vi "sine_wave_generator.vi"(7 "Source":T1={"Source"=TRUE, "Source type"=FALSE, "Amplitude"=1.0, "Period"=100.0} {"Amplitude" scale=0.0..1.0; "Period" scale=1.0..1000.0}) -> (8 "Output":dbl)   [LabVIEW 2016]
doc: "Use this VI to generate sine wave.\n\nInputs:\nSource (typedef).\nOutputs:\nOutput.\n\nMuhannad Alghamdi\nCSUSB Physics 350"
uses:
  typedefs/periodic_signal_control.ctl
panel:
  out "Call counter":dbl
  # "Sine Wave Generator"
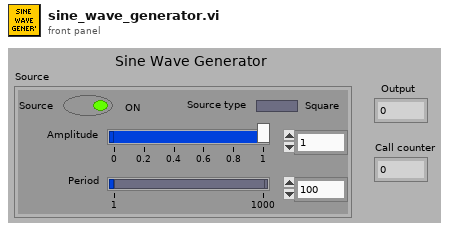
[diagram p1: front panel]
types:
  T1 = typedef "periodic_signal_control.ctl" = cluster{"Source":bool, "Source type":bool, "Amplitude":dbl, "Period":dbl}
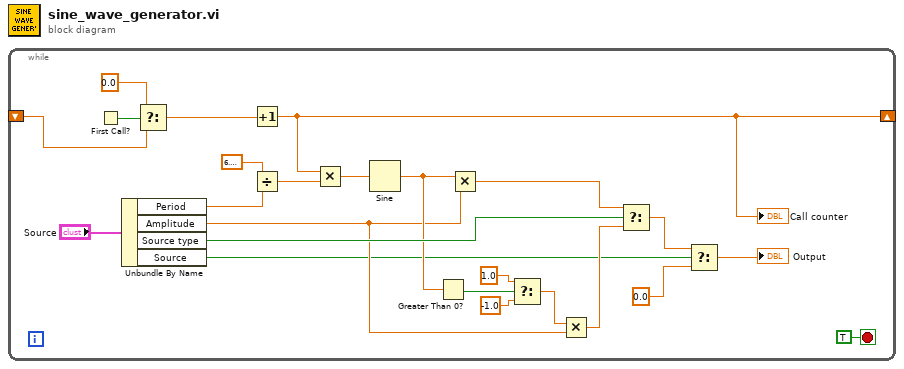
[diagram p0: block diagram]
diagram:
  n1 = while {
    shift-right: [w1] -> _
    shift-left: _ -> [w21]
    stop <- TRUE stop-if-true
    n2 = First Call?() -> (First Call?: T/F=w22:bool)
    n3 = Unbundle By Name("Source") -> ("Period"=w15:dbl, "Amplitude"=w8:dbl, "Source type"=w13:bool, "Source"=w4:bool)
    n4 = Select(t=0.0, s=w22, f=w21) -> (s? t:f=w23:dbl)
    n5 = Increment(x=w23) -> (x+1=w1:dbl)
    "Call counter" <- w1
    n6 = Divide(x=6.283185307179586, y=w15) -> (x/y=w17:dbl)
    n7 = Multiply(x=w1, y=w17) -> (x*y=w18:dbl)
    n8 = Sine(x=w18) -> (sin(x)=w12:dbl)
    n9 = Greater Than 0?(x=w12) -> (x > 0?=w2:bool)
    n10 = Multiply(x=w12, y=w8) -> (x*y=w14:dbl)
    n11 = Select(t=1.0, s=w2, f=-1.0) -> (s? t:f=w9:dbl)
    n12 = Multiply(x=w9, y=w8) -> (x*y=w7:dbl)
    n13 = Select(t=w14, s=w13, f=w7) -> (s? t:f=w6:dbl)
    n14 = Select(t=w6, s=w4, f=0.0) -> (s? t:f=→"Output":dbl)
  }
